vi "TemperatureMeasure.vi"(4 "低温？":bool, 5 "error in":errorcluster, 6 "Color Image":T1, 7 "Gray Image":T1, 8 "On/Off":bool) -> (0 "error out":errorcluster, 1 "温度分布簇":cluster{dbl[], i32[]}, 2 "实时温度":T2, 3 "平均温度":dbl format="%0.2f")   [LabVIEW 2012]
uses:
  <vilib>/vision/Image Controls.llb/IMAQ Image.ctl
  <vilib>/Analysis/baseanly.llb/Unimode.vi
  <vilib>/vision/NI_Vision_Development_Module.lvlib
  <vilib>/Analysis/NI_AALBase.lvlib
  <vilib>/gmath/NI_Gmath.lvlib
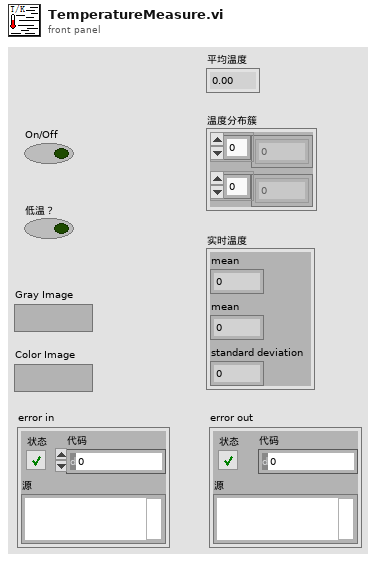
[diagram p1: front panel]
types:
  T1 = typedef "IMAQ Image.ctl" = refnum<image>
  T2 = cluster{"mean":dbl, "mean":dbl, "standard deviation":dbl}
  T3 = typedef "Image Type" = u32
  T4 = cluster{"mode":dbl, "mode":dbl, "spread value":dbl}
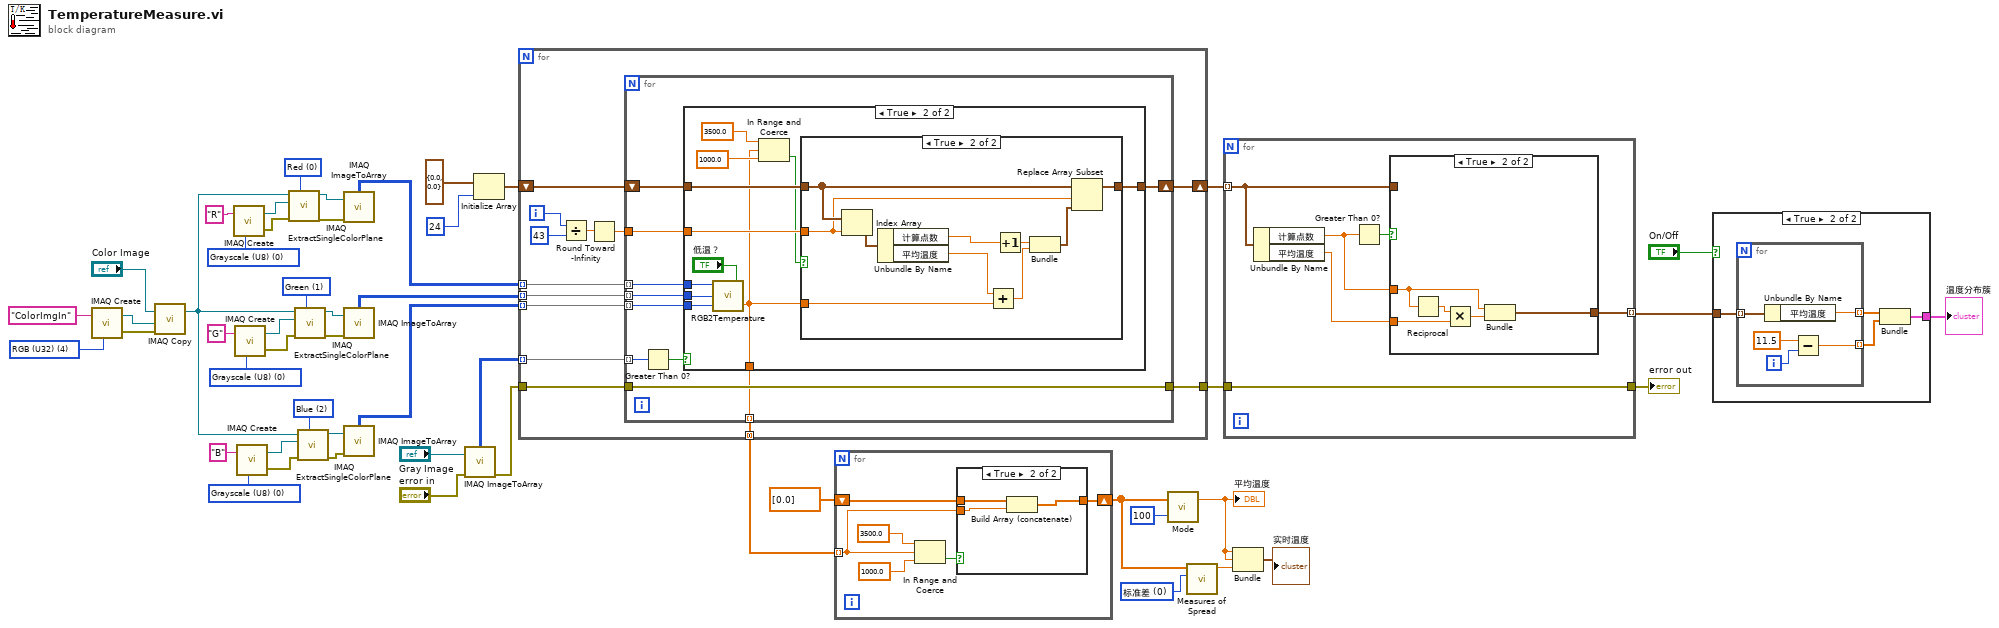
[diagram p0: block diagram]
diagram:
  w5 = 0 items=["标准差", "范围", "均值绝对偏差", "四分位数间距"] ("type")
  w20 = T3 0 items=["Grayscale (U8)", "Grayscale (I16)", "Grayscale (SGL)", "Complex (CSG)", "RGB (U32)", "HSL (U32)", "RGB (U64)", "Grayscale (U16)"] ("Image Type")
  w21 = T3 0 items=["Grayscale (U8)", "Grayscale (I16)", "Grayscale (SGL)", "Complex (CSG)", "RGB (U32)", "HSL (U32)", "RGB (U64)", "Grayscale (U16)"] ("Image Type")
  w22 = T3 0 items=["Grayscale (U8)", "Grayscale (I16)", "Grayscale (SGL)", "Complex (CSG)", "RGB (U32)", "HSL (U32)", "RGB (U64)", "Grayscale (U16)"] ("Image Type")
  w34 = 2 items=["Red", "Green", "Blue", "Hue", "Saturation", "Luminance", "Value", "Intensity"] ("Color Plane")
  w35 = 1 items=["Red", "Green", "Blue", "Hue", "Saturation", "Luminance", "Value", "Intensity"] ("Color Plane")
  w36 = 0 items=["Red", "Green", "Blue", "Hue", "Saturation", "Luminance", "Value", "Intensity"] ("Color Plane")
  w47 = T3 4 items=["Grayscale (U8)", "Grayscale (I16)", "Grayscale (SGL)", "Complex (CSG)", "RGB (U32)", "HSL (U32)", "RGB (U64)", "Grayscale (U16)"] ("Image Type")
  n1 = call "IMAQ Create"("Image Name"="ColorImgIn", "Image Type"=w47) -> ("New Image"=w40:T1, "error out"=w41:errorcluster)  [unwired: 3 in]
  n2 = call "IMAQ Copy"("error in (no error)"=w41, "Image Dst"=w40, "Image Src"="Color Image") -> ("Image Dst Out"=w12:T1)  [unwired: 3 in, 1 out]
  n3 = call "IMAQ Create"("Image Name"="R", "Image Type"=w21) -> ("New Image"=w31:T1, "error out"=w25:errorcluster)  [unwired: 3 in]
  n4 = call "IMAQ Create"("Image Name"="G", "Image Type"=w20) -> ("New Image"=w32:T1, "error out"=w24:errorcluster)  [unwired: 3 in]
  n5 = call "IMAQ Create"("Image Name"="B", "Image Type"=w22) -> ("New Image"=w33:T1, "error out"=w23:errorcluster)  [unwired: 3 in]
  n6 = call "IMAQ ExtractSingleColorPlane"("Color Plane"=w36, "error in (no error)"=w25, "Image Dst"=w31, "Image Src"=w12) -> ("error out"=w26:errorcluster, "Image Dst Out"=w27:T1)  [unwired: 6 in]
  n7 = call "IMAQ ExtractSingleColorPlane"("Color Plane"=w35, "error in (no error)"=w24, "Image Dst"=w32, "Image Src"=w12) -> ("error out"=w18:errorcluster, "Image Dst Out"=w19:T1)  [unwired: 6 in]
  n8 = call "IMAQ ExtractSingleColorPlane"("Color Plane"=w34, "error in (no error)"=w23, "Image Dst"=w33, "Image Src"=w12) -> ("error out"=w16:errorcluster, "Image Dst Out"=w17:T1)  [unwired: 6 in]
  n9 = call "IMAQ ImageToArray"("error in (no error)"=w26, "Image"=w27) -> ("Image Pixels (U8)"=w44:u8[][])  [unwired: 2 in, 4 out]
  n10 = call "IMAQ ImageToArray"("error in (no error)"=w18, "Image"=w19) -> ("Image Pixels (U8)"=w43:u8[][])  [unwired: 2 in, 4 out]
  n11 = call "IMAQ ImageToArray"("error in (no error)"=w16, "Image"=w17) -> ("Image Pixels (U8)"=w42:u8[][])  [unwired: 2 in, 4 out]
  n12 = call "IMAQ ImageToArray"("error in (no error)"="error in", "Image"="Gray Image") -> ("error out"=w30:errorcluster, "Image Pixels (U8)"=w8:u8[][])  [unwired: 2 in, 3 out]
  n13 = Initialize Array(cluster{"计算点数":dbl, "平均温度":dbl} {"计算点数"=0.0, "平均温度"=0.0} ("温度信号簇"), 24 ("维数大小")) -> (w51:cluster{"计算点数":dbl, "平均温度":dbl}[])
  n14 = for {
    tunnel: w8 -> [w64] mode=indexing
    shift-right: [w60] -> w46
    shift-left: w51 -> [w61]
    tunnel: w44 -> [w58] mode=indexing
    tunnel: w43 -> [w57] mode=indexing
    tunnel: w42 -> [w56] mode=indexing
    tunnel: w30 -> [w53]
    tunnel: [w54] -> w29
    tunnel: [w52] -> w6 mode=concatenating
    i -> [w59]
    n15 = Divide(x=w59, y=43) -> (x/y=w62:dbl)
    n16 = Round Toward -Infinity(1:w62) -> (0:w55:dbl)
    n17 = for {
      tunnel: w64 -> [w74] mode=indexing
      shift-right: [w71] -> w60
      shift-left: w61 -> [w72]
      tunnel: w58 -> [w70] mode=indexing
      tunnel: w57 -> [w69] mode=indexing
      tunnel: w56 -> [w68] mode=indexing
      tunnel: w55 -> [w67]
      tunnel: [w66] -> w54
      tunnel: w53 -> [w66]
      tunnel: [w65] -> w52 mode=indexing
      n18 = Greater Than 0?(x=w74) -> (x > 0?=w73:bool)
      n19 = case shown="True" w73 {
        tunnel: w69 -> [_ w82]
        tunnel: w70 -> [_ w81]
        tunnel: w68 -> [_ w83]
        tunnel: [w75 w86] -> w71
        tunnel: w72 -> [w75 w85]
        tunnel: w67 -> [_ w84]
        tunnel: [_ w77] -> w65
        frame False {
        }
        frame True {
          n20 = call "RGB2Temperature.vi"("低温？"="低温？", "B"=w83, "G"=w82, "R"=w81) -> ("Temperature"=w77:dbl)
          n21 = In Range and Coerce(upper limit=3500.0 ("上限"), x=w77, lower limit=1000.0 ("下限")) -> (In Range?=w76:bool)  [unwired: 1 out]
          n22 = case shown="True" w76 {
            tunnel: [w87 w97] -> w86
            tunnel: w85 -> [w87 w96]
            tunnel: w84 -> [_ w89]
            tunnel: w77 -> [_ w88]
            frame False {
            }
            frame True {
              n23 = Index Array(array=w96, index=w89) -> (element=w95:cluster{"计算点数":dbl, "平均温度":dbl})
              n24 = Unbundle By Name(w95) -> ("计算点数"=w93:dbl, "平均温度"=w94:dbl)
              n25 = Add(x=w94, y=w88) -> (x+y=w91:dbl)
              n26 = Increment(x=w93) -> (x+1=w92:dbl)
              n27 = Bundle(w92, w91) -> (w90:cluster{dbl, dbl})  [unwired: 1 in]
              n28 = Replace Array Subset(array=w96, new element=w90, index=w89) -> (w97:cluster{"计算点数":dbl, "平均温度":dbl}[])
            }
          }
        }
      }
    }
  }
  n29 = for {
    shift-right: [w102] -> w3
    shift-left: dbl[] [0.0] -> [w103]
    tunnel: w6 -> [w101] mode=indexing
    n30 = In Range and Coerce(upper limit=3500.0 ("上限"), x=w101, lower limit=1000.0 ("下限")) -> (In Range?=w100:bool)  [unwired: 1 out]
    n31 = case shown="True" w100 {
      tunnel: w103 -> [w104 w107]
      tunnel: w101 -> [_ w106]
      tunnel: [w104 w105] -> w102
      frame False {
      }
      frame True {
        n32 = Build Array (concatenate)(w107, w106) -> (w105:dbl[])
      }
    }
  }
  n33 = call-poly <vilib>:"Mode.vi"("intervals"=100, "X"=w3) -> ("mode"=w2:dbl)  [unwired: 1 out]
  "平均温度" <- w2
  n34 = call <vilib>:"Measures of Spread.vi"("type"=w5, "x array"=w3) -> ("spread value"=w4:dbl)  [unwired: 8 in, 1 out]
  n35 = for {
    tunnel: w46 -> [w113] mode=indexing
    tunnel: [w109] -> w14 mode=indexing
    tunnel: [w108] -> w28
    tunnel: w29 -> [w108]
    n36 = Unbundle By Name(w113) -> ("计算点数"=w111:dbl, "平均温度"=w110:dbl)
    n37 = Greater Than 0?(x=w111) -> (x > 0?=w112:bool)
    n38 = case shown="True" w112 {
      tunnel: w113 -> [w114 _]
      tunnel: w111 -> [_ w116]
      tunnel: w110 -> [_ w118]
      tunnel: [w114 w115] -> w109
      frame False {
      }
      frame True {
        n39 = Reciprocal(x=w116) -> (1/x=w119:dbl)
        n40 = Multiply(x=w119, y=w118) -> (x*y=w117:dbl)
        n41 = Bundle("计算点数"=w116, w117) -> (w115:cluster{"计算点数":dbl, dbl})  [unwired: 1 in]
      }
    }
  }
  "error out" <- w28
  n42 = Bundle("mode"=w2, "mode"=w2, "spread value"=w4) -> (→"实时温度":T4)  [unwired: 1 in]
  n43 = case shown="True" "On/Off" {
    tunnel: [_ w121] -> w15
    tunnel: w14 -> [_ w120]
    frame False {
    }
    frame True {
      n44 = for {
        tunnel: w120 -> [w128] mode=indexing
        tunnel: [w127] -> w122 mode=indexing
        tunnel: [w124] -> w123 mode=indexing
        i -> [w126]
        n45 = Unbundle By Name(w128) -> ("平均温度"=w127:dbl)
        n46 = Subtract(x=11.5, y=w126) -> (x-y=w124:dbl)
      }
      n47 = Bundle(w122, w123) -> (w121:cluster{dbl[], dbl[]})  [unwired: 1 in]
    }
  }
  "温度分布簇" <- w15
